vi "VisualizePmuResults.vi"() -> ()   [LabVIEW 2018, in "Visualization.lvlib" / "VisualizeAnalysis.lvclass"]
uses:
  VisualizeAnalysis.lvclass
  VisualizeBase/VisualizeBase_class/Requests/clUserEventType.ctl
  <vilib>/event_ctls.llb/usereventprio.ctl
  <vilib>/Utility/file.llb/Read From Spreadsheet File (DBL).vi
  <vilib>/Utility/error.llb/Error Cluster From Error Code.vi
  <vilib>/ErrorRing/Error Ring.xnode
  VisualizeBase/VisualizeBase_class/VisualizeBase.lvclass
  <userlib>/NIST/NISTErrorLib/NISTErrorLib.lvlib
  Analysis/AnalysisModule/AnalysisModule.lvlib
panel:
  in  "btnReset":bool
  in  "btnClear":bool
  in  "Pause":bool
  out "Data from file":dbl[][](array[numeric])
  in  "btnOpen":bool
  out "RFE":dbl(graph)
  out "FE":dbl(graph)
  out "Data real time":dbl[](array[numeric])
  out "TVE":cluster{timestamp[], dbl[]}[](graph)
  in  "QueName":string="AnalVisQue"
  out "ErrorArray":errorcluster[](array[cluster])
  in  "btnStop":bool
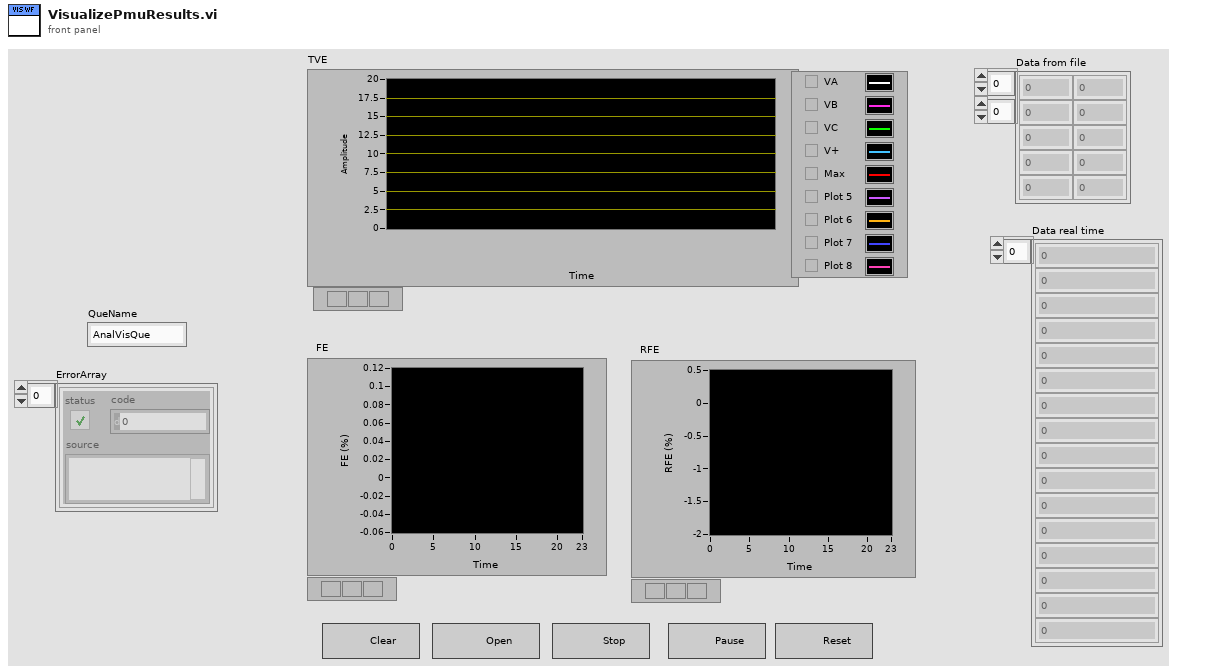
[diagram p1: front panel]
types:
  T1 = typedef "Visualization.lvlib/VisualizeBase.lvclass/clRequestEvents.ctl" = cluster{"StopRequest":refnum<user-event>, "ResetRequest":refnum<user-event>}
  T2 = typedef "AnalysisModule.lvlib/clBroadcastEvents.ctl" = cluster{"DidInit":refnum<user-event>, "StatusUpdate":refnum<user-event>, "ErrorReport":refnum<user-event>, "DidStop":refnum<user-event>, "PathToINI":refnum<user-event>, "Config":refnum<user-event>, "ResultReport":refnum<user-event>, "FunctionClass":refnum<user-event>}
  T3 = typedef "Visualization.lvlib/VisualizeBase.lvclass/clUserEventType.ctl" = cluster{"BusIndex":i8, "Data":variant}
  T4 = typedef "usereventprio.ctl" = enum32{"high priority", "normal priority"}
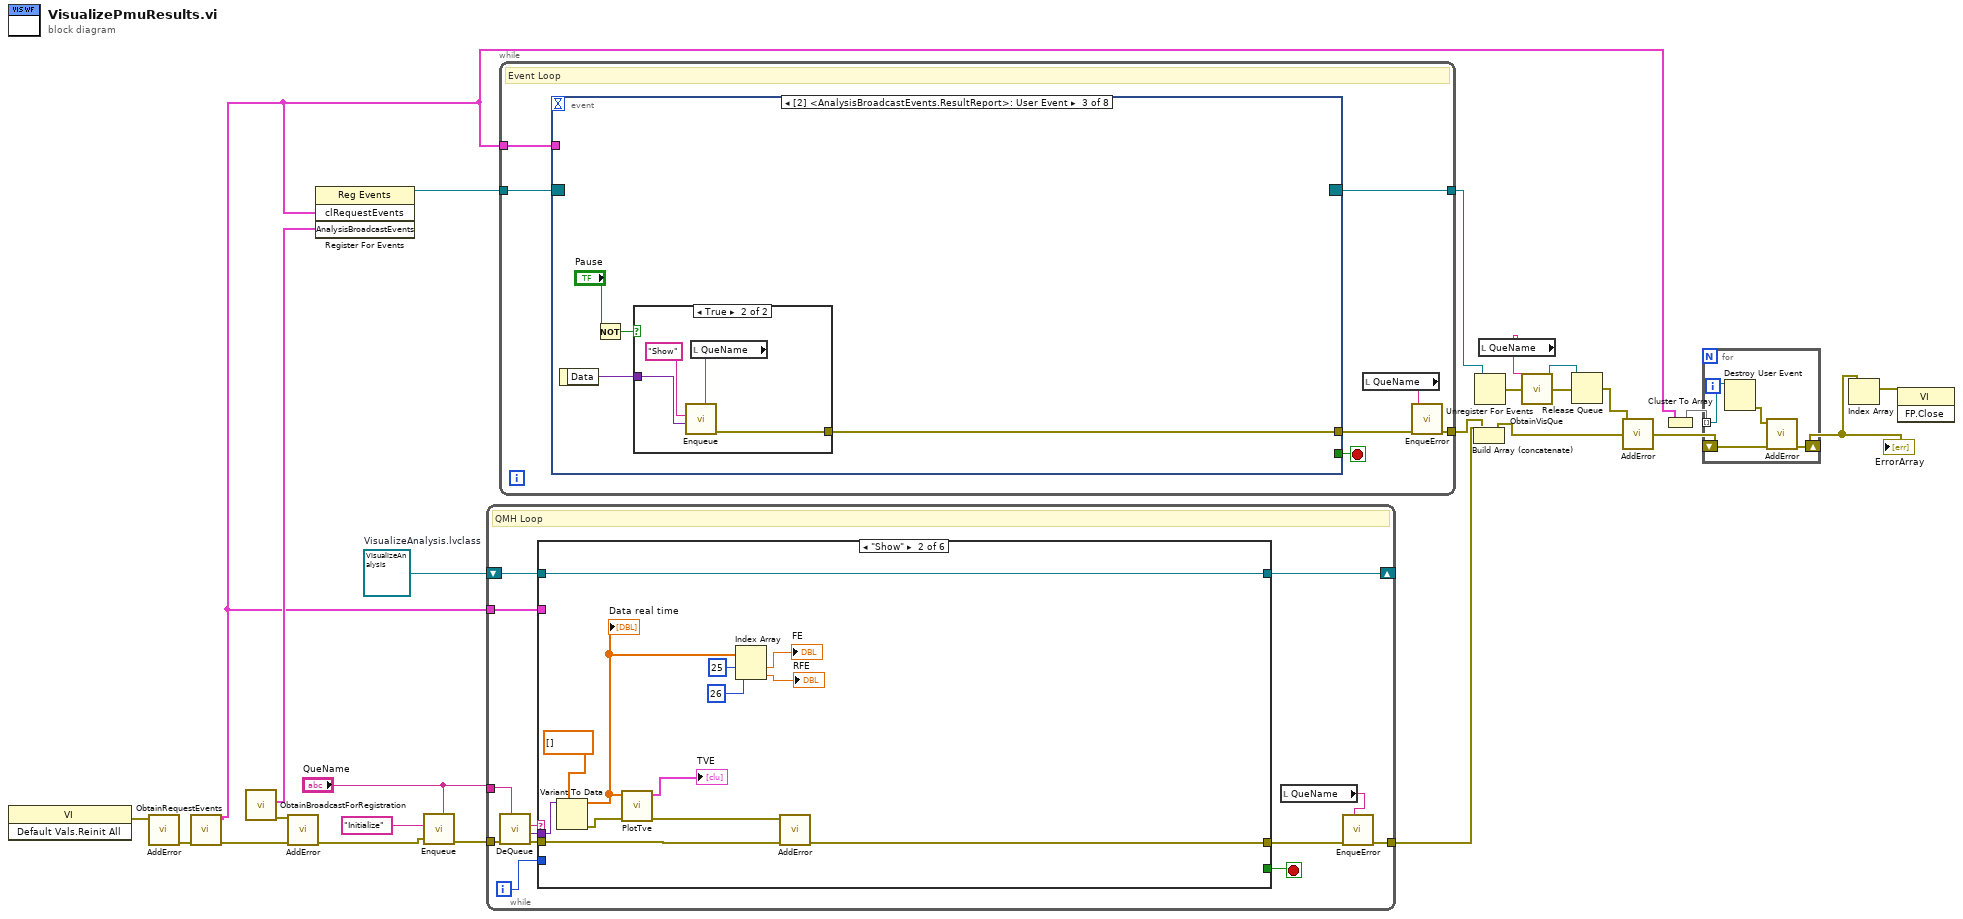
[diagram p0: block diagram]
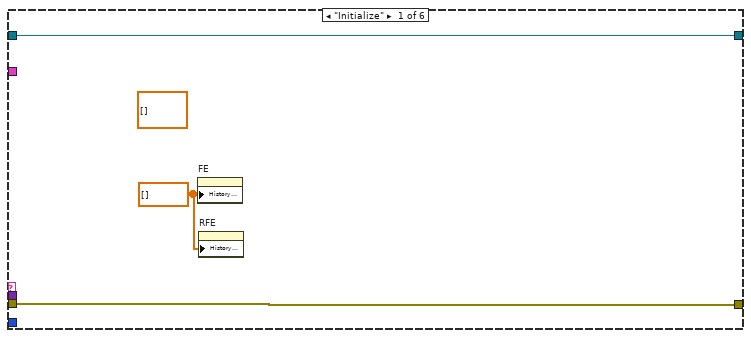
[diagram p2: hidden frame]
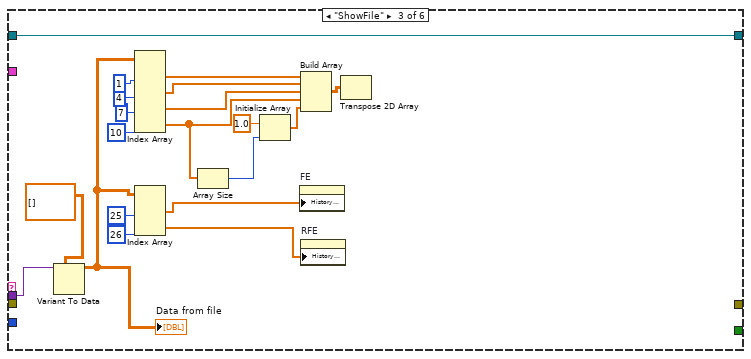
[diagram p3: hidden frame]
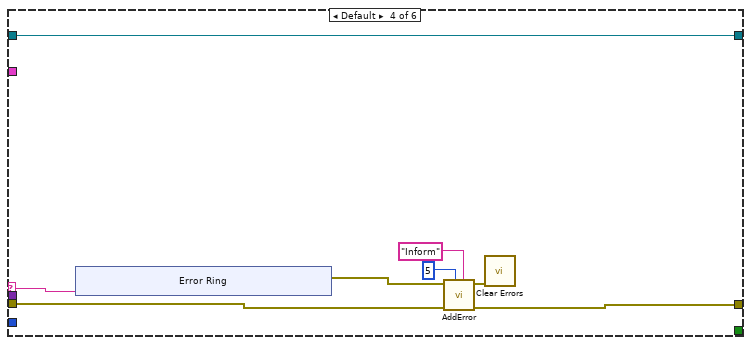
[diagram p4: hidden frame]
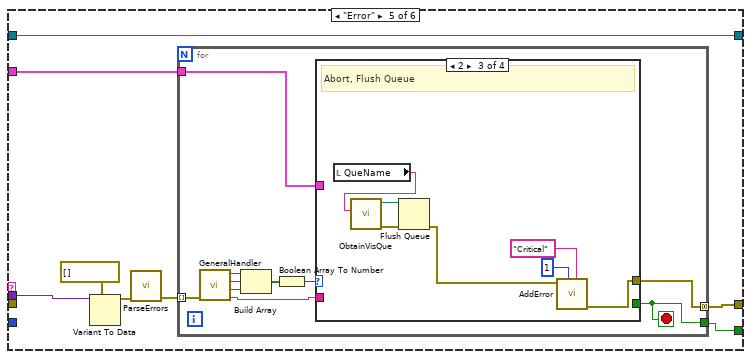
[diagram p5: hidden frame]
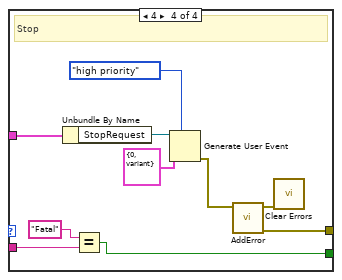
[diagram p8: hidden frame]
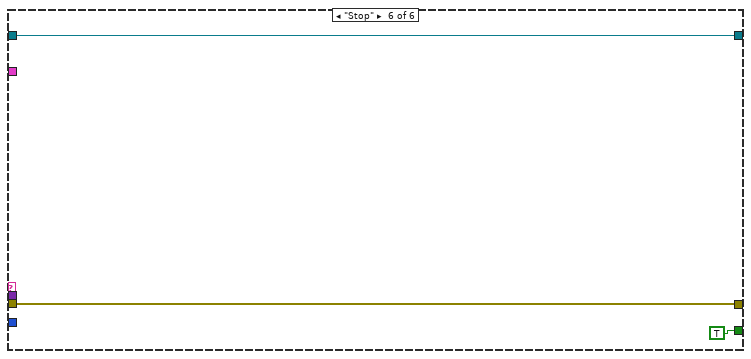
[diagram p9: hidden frame]
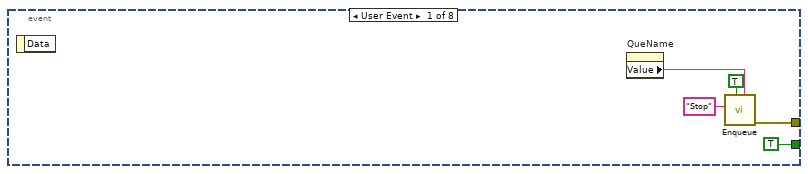
[diagram p10: hidden frame]
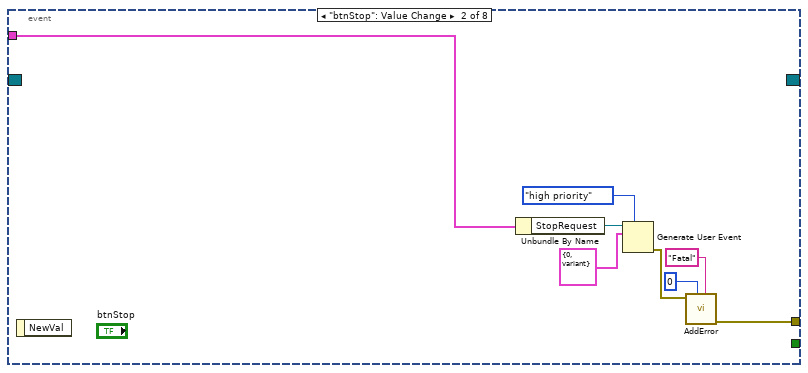
[diagram p11: hidden frame]
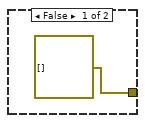
[diagram p12: hidden frame]
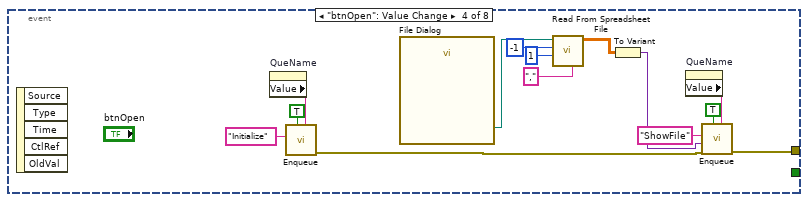
[diagram p13: hidden frame]
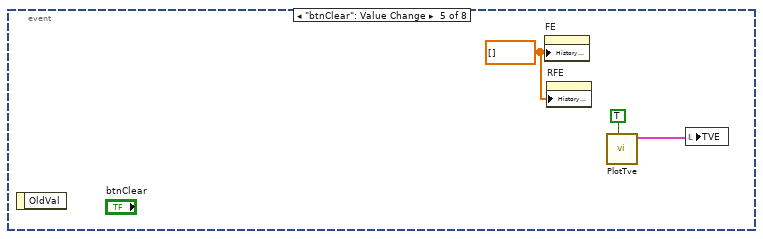
[diagram p14: hidden frame]
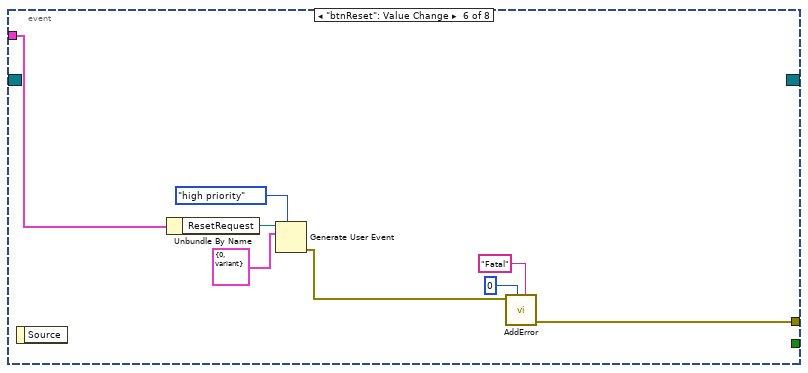
[diagram p15: hidden frame]
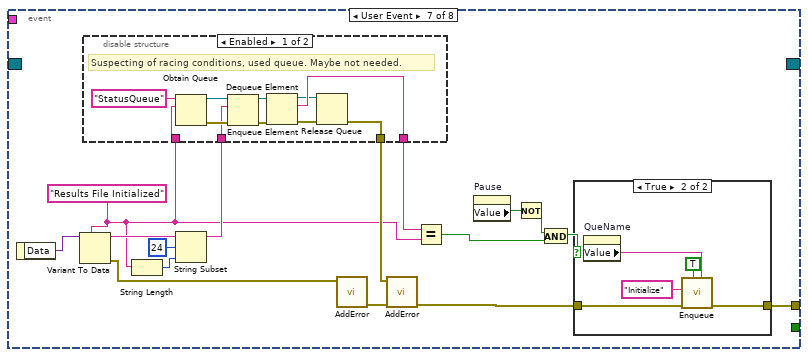
[diagram p16: hidden frame]
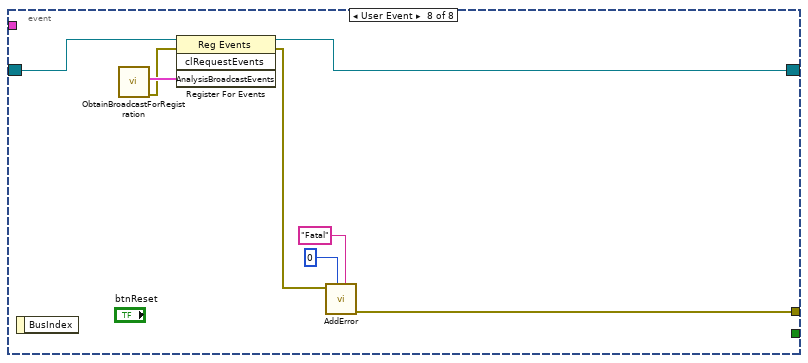
[diagram p19: hidden frame]
diagram:
  w14 = refnum<class "VisualizeAnalysis.lvclass"> refnum  # VisualizeAnalysis.lvclass
  n1 = invoke class="VI" method="Default Vals.Reinit All"() -> (error out=w21:errorcluster)  [unwired: 3 in, 2 out]
  n2 = call <userlib>:"AddError.vi"("error in (no error)"=w21) -> ("ErrorArray"=w20:errorcluster[])  [unwired: 9 in, 1 out]
  n3 = call "ObtainRequestEvents.vi"("Error"=w20) -> ("Error"=w18:errorcluster[], "clRequestEvents"=w1:T1)  [unwired: 9 in]
  n4 = call "ObtainBroadcastForRegistration.vi"() -> ("error out"=w16:errorcluster, "AnalysisBroadcastEvents"=w19:T2)  [unwired: 10 in]
  n5 = call <userlib>:"AddError.vi"("ErrorArray"=w18, "error in (no error)"=w16) -> ("ErrorArray"=w17:errorcluster[])  [unwired: 8 in, 1 out]
  n6 = register-events(w1, w19) -> (reference out=w13:refnum<event-registration>)  [unwired: 2 in, 1 out]
  n7 = call "Enqueue.vi"("QueName"="QueName", "Error"=w17, "Message"="Initialize") -> ("Error"=w24:errorcluster[])  [unwired: 8 in]
  n8 = while {
    tunnel: w24 -> [w38]
    tunnel: [w32] -> w23
    tunnel: "QueName" -> [w30]
    shift-right: [w29] -> _
    shift-left: w14 -> [w28]
    tunnel: w1 -> [w27]
    i -> [w26]
    stop <- w33 stop-if-true
    # "QMH Loop"
    n9 = call "DeQueue.vi"("QueName"=w30, "Error"=w38) -> ("Error"=w35:errorcluster[], "Data"=w36:variant, "Message"=w37:string)  [unwired: 7 in]
    n10 = case shown="\"Show\"" w37 {
      selector: w37 -> [_ _ _ w82 _ _]
      tunnel: w36 -> [_ w53 w74 _ w97 _]
      tunnel: w35 -> [w41 w48 _ w80 _ w126]
      tunnel: [w41 w47 _ w79 w93 w126] -> w34
      tunnel: [_ _ _ _ w92 TRUE] -> w33
      tunnel: w28 -> [w40 w54 w72 w75 w91 w125]
      tunnel: [w40 w54 w72 w75 w91 w125] -> w29
      tunnel: w27 -> [_ _ _ _ w90 _]
      tunnel: w26 -> [_ _ _ _ _ _]
      frame "Initialize" {
        w39 = dbl[] [] ("History Data")
        (unwired) dbl[][] [] ("History Data")
        n11 = property on="FE" class="WFChart (strict)"("History Data"=w39) -> ()  [unwired: 2 in, 2 out]
        n12 = property on="RFE" class="WFChart (strict)"("History Data"=w39) -> ()  [unwired: 2 in, 2 out]
      }
      frame "Show" {
        n13 = Variant To Data(type=dbl[] [], Variant=w53) -> (data=w44:dbl[], error out=w46:errorcluster)  [unwired: 1 in]
        "Data real time" <- w44
        n14 = call "PlotTve.vi"("error in (no error)"=w46, "Data real time"=w44) -> ("error out"=w45:errorcluster, "TVE"=→"TVE":cluster{timestamp[], dbl[]}[])  [unwired: 8 in]
        n15 = Index Array(array=w44, index #1=25 ("index"), index #2=26 ("index")) -> (element #1=→"FE":dbl, element #2=→"RFE":dbl)
        n16 = call <userlib>:"AddError.vi"("ErrorArray"=w48, "error in (no error)"=w45) -> ("ErrorArray"=w47:errorcluster[])  [unwired: 8 in, 1 out]
      }
      frame "ShowFile" {
        n17 = Variant To Data(type=dbl[][] [], Variant=w74) -> (data=w63:dbl[][])  [unwired: 1 in, 1 out]
        "Data from file" <- w63
        n18 = Index Array(array=w63, index (col) #1=1 ("disabled index (col)"), index (col) #2=4 ("index (col)"), index (col) #3=7 ("index (col)"), index (col) #4=10 ("index (col)")) -> (element #1=w67:dbl[], element #2=w66:dbl[], element #3=w65:dbl[], element #4=w58:dbl[])  [unwired: 4 in]
        n19 = Index Array(array=w63, index (col) #1=25 ("disabled index (col)"), index (col) #2=26 ("index (col)")) -> (element #1=w60:dbl[], element #2=w59:dbl[])  [unwired: 2 in]
        n20 = Array Size(array=w58) -> (size(s)=w57:i32)
        n21 = Initialize Array(1.0 ("element"), w57) -> (w55:dbl[])
        n22 = property on="FE" class="WFChart (strict)"("History Data"=w60) -> ()  [unwired: 2 in, 2 out]
        n23 = Build Array(w67, w66, w65, w58, w55) -> (w64:dbl[][])
        n24 = property on="RFE" class="WFChart (strict)"("History Data"=w59) -> ()  [unwired: 2 in, 2 out]
        n25 = Transpose 2D Array(2D array=w64) -> ()  [unwired: 1 out]
      }
      frame Default {
        n26 = xnode "Error Ring"("parameter 0"=w82) -> ("error out"=w81:errorcluster)
        n27 = call <userlib>:"AddError.vi"("Severity"="Inform" ("String"), "Priority"=u8 5, "ErrorArray"=w80, "error in (no error)"=w81) -> ("ErrorArray"=w79:errorcluster[], "error out"=w78:errorcluster)  [unwired: 6 in]
        n28 = call <vilib>:"Clear Errors.vi"("error in (no error)"=w78) -> ()  [unwired: 5 in, 2 out]
      }
      frame "Error" {
        n29 = Variant To Data(type=errorcluster[] [], Variant=w97) -> (data=w95:errorcluster[])  [unwired: 1 in, 1 out]
        n30 = call <userlib>:"ParseErrors.vi"("ErrorArray"=w95) -> ("ErrorArray"=w94:errorcluster[])  [unwired: 8 in, 2 out]
        n31 = for {
          tunnel: w94 -> [w107] mode=indexing
          tunnel: [w101] -> w93 mode=concatenating
          tunnel: [w99] -> w92
          tunnel: w90 -> [w98]
          stop <- w99 stop-if-true
          n32 = call <userlib>:"GeneralHandler.vi"("error in (no error)"=w107) -> ("Severity"=w100:string, "Stop"=w104:bool, "Abort"=w105:bool, "Continue"=w106:bool)  [unwired: 7 in]
          n33 = Build Array(w106, w105, w104) -> (w103:bool[])
          n34 = Boolean Array To Number(Boolean array=w103) -> (number=w102:u32)
          n35 = case shown="2" w102 {
            tunnel: [_ _ w112 w123] -> w101
            tunnel: w100 -> [_ _ _ w118]
            tunnel: [_ _ _ w116] -> w99
            tunnel: w98 -> [_ _ _ w115]
            frame 0, Default {
              # "No Dialog"
            }
            frame 1 {
              # "Continue"
            }
            frame 2 {
              # "Abort, Flush Queue"
              n36 = local read "QueName"() -> (w108:string)
              n37 = call "ObtainVisQue.vi"("QueName"=w108) -> ("error out"=w114:errorcluster, "queue out"=w113:refnum<queue>)  [unwired: 9 in]
              n38 = Flush Queue(queue=w113, error in (no error)=w114) -> (error out=w111:errorcluster)  [unwired: 2 out]
              n39 = call <userlib>:"AddError.vi"("Severity"="Critical" ("String"), "Priority"=u8 1, "error in (no error)"=w111) -> ("ErrorArray"=w112:errorcluster[])  [unwired: 7 in, 1 out]
            }
            frame 4 {
              # "Stop"
              n40 = Unbundle By Name(w115) -> ("StopRequest"=w124:refnum<user-event>)
              n41 = Equal?(x="Fatal", y=w118) -> (x = y?=w116:bool)
              n42 = Generate User Event(priority (normal)=usereventprio."high priority", user event=w124, event data cluster=T3 {"BusIndex"=0, "Data"=variant} ("event data")) -> (error out=w122:errorcluster)  [unwired: 1 in, 1 out]
              n43 = call <userlib>:"AddError.vi"("error in (no error)"=w122) -> ("ErrorArray"=w123:errorcluster[], "error out"=w119:errorcluster)  [unwired: 9 in]
              n44 = call <vilib>:"Clear Errors.vi"("error in (no error)"=w119) -> ()  [unwired: 5 in, 2 out]
            }
          }
        }
      }
      frame "Stop" {
      }
    }
    n45 = local read "QueName"() -> (w31:string)
    n46 = call "EnqueError.vi"("QueName"=w31, "Error"=w34) -> ("Error"=w32:errorcluster[])  [unwired: 9 in]
  }
  n47 = while {
    tunnel: [w132] -> w22
    tunnel: w13 -> [w130]
    tunnel: [w129] -> w7
    tunnel: w1 -> [w128]
    stop <- w134 stop-if-true
    # "Event Loop"
    n48 = event shown="[2] <AnalysisBroadcastEvents.ResultReport>: User Event" {
      selector: w130 -> [_ _ _ _ _ _ _ w216]
      dyn-events: [_ _ _ _ _ _ _ w221] -> w129
      timeout: _ -> [_ _ _ _ _ _ _ _]
      tunnel: [TRUE _ _ _ _ _ _ _] -> w134
      tunnel: [w138 w145 w150 w165 _ w174 w196 w217] -> w133
      tunnel: w128 -> [_ w140 _ _ _ w175 _ _]
      event User Event {
        n49 = event-data() -> ()  [unwired: 1 in, 1 out]
        n50 = property on="QueName" class="Str"() -> ("Value"=w135:string)  [unwired: 2 in, 2 out]
        n51 = call "Enqueue.vi"("QueName"=w135, "Priority? (F)"=TRUE, "Message"="Stop") -> ("Error"=w138:errorcluster[])  [unwired: 8 in]
      }
      event "btnStop": Value Change {
        n52 = event-data() -> ()  [unwired: 1 in, 1 out]
        n53 = Unbundle By Name(w140) -> ("StopRequest"=w146:refnum<user-event>)
        n54 = Generate User Event(priority (normal)=usereventprio."high priority", user event=w146, event data cluster=T3 {"BusIndex"=0, "Data"=variant} ("event data")) -> (error out=w147:errorcluster)  [unwired: 1 in, 1 out]
        n55 = call <userlib>:"AddError.vi"("Severity"="Fatal" ("String"), "Priority"=u8 0, "error in (no error)"=w147) -> ("ErrorArray"=w145:errorcluster[])  [unwired: 7 in, 1 out]
      }
      event User Event {
        n56 = event-data() -> ("Data"=w151:variant)  [unwired: 1 in]
        n57 = Not(x="Pause") -> (.not. x?=w148:bool)
        n58 = case shown="True" w148 {
          tunnel: w151 -> [_ w155]
          tunnel: [errorcluster[] [] ("Error") w154] -> w150
          frame False {
          }
          frame True {
            n59 = local read "QueName"() -> (w156:string)
            n60 = call "Enqueue.vi"("QueName"=w156, "Data"=w155, "Message"="Show") -> ("Error"=w154:errorcluster[])  [unwired: 8 in]
          }
        }
      }
      event "btnOpen": Value Change {
        n61 = event-data() -> ()  [unwired: 1 in, 5 out]
        n62 = property on="QueName" class="Str"() -> ("Value"=w162:string)  [unwired: 2 in, 2 out]
        n63 = call "Enqueue.vi"("QueName"=w162, "Priority? (F)"=TRUE, "Message"="Initialize") -> ("Error"=w159:errorcluster[])  [unwired: 8 in]
        n64 = call "File Dialog"() -> ("selected path"=w170:path)  [unwired: 12 in, 3 out]
        n65 = call-poly <vilib>:"Read From Spreadsheet File.vi"("delimiter (\\t)"="," ("delimiter (\\t)"), "start of read offset (chars.:0)"=1, "number of rows (all:-1)"=-1, "file path (dialog if empty)"=w170) -> ("all rows"=w164:dbl[][])  [unwired: 3 in, 4 out]
        n66 = To Variant(anything=w164) -> (Variant=w163:variant)
        n67 = property on="QueName" class="Str"() -> ("Value"=w166:string)  [unwired: 2 in, 2 out]
        n68 = call "Enqueue.vi"("QueName"=w166, "Priority? (F)"=TRUE, "Error"=w159, "Data"=w163, "Message"="ShowFile") -> ("Error"=w165:errorcluster[])  [unwired: 6 in]
      }
      event "btnClear": Value Change {
        w171 = dbl[] [] ("History Data")
        n69 = event-data() -> ()  [unwired: 1 in, 1 out]
        n70 = property on="FE" class="WFChart (strict)"("History Data"=w171) -> ()  [unwired: 2 in, 2 out]
        n71 = property on="RFE" class="WFChart (strict)"("History Data"=w171) -> ()  [unwired: 2 in, 2 out]
        n72 = call "PlotTve.vi"("Clear? (f)"=TRUE) -> ("TVE"=w172:cluster{timestamp[], dbl[]}[])  [unwired: 9 in, 1 out]
        n73 = local write "TVE"(w172) -> ()
      }
      event "btnReset": Value Change {
        n74 = event-data() -> ()  [unwired: 1 in, 1 out]
        n75 = Unbundle By Name(w175) -> ("ResetRequest"=w176:refnum<user-event>)
        n76 = Generate User Event(priority (normal)=usereventprio."high priority", user event=w176, event data cluster=T3 {"BusIndex"=0, "Data"=variant} ("event data")) -> (error out=w179:errorcluster)  [unwired: 1 in, 1 out]
        n77 = call <userlib>:"AddError.vi"("Severity"="Fatal", "Priority"=u8 0, "error in (no error)"=w179) -> ("ErrorArray"=w174:errorcluster[])  [unwired: 7 in, 1 out]
      }
      event User Event {
        w186 = "Results File Initialized" ("Status")
        n78 = event-data() -> ("Data"=w197:variant)  [unwired: 1 in]
        n79 = Variant To Data(type=w186, Variant=w197) -> (data=w194:string, error out=w191:errorcluster)  [unwired: 1 in]
        n80 = String Length(string=w186) -> (length=w187:i32)
        n81 = String Subset(string=w194, offset (0)=24, length (rest)=w187) -> (substring=w189:string)
        n82 = disable-structure shown="Enabled" {
          disable-tunnel: [w201 w209] -> w193
          disable-tunnel: [w198 _] -> w190
          disable-tunnel: w189 -> [w203 w209]
          disable-tunnel: w186 -> [w202 _]
          frame Enabled {
            # "Suspecting of racing conditions, used queue. Maybe not needed."
            n83 = Obtain Queue(name (unnamed)="StatusQueue", element data type=w202) -> (queue out=w207:refnum<queue>, error out=w205:errorcluster)  [unwired: 3 in, 1 out]
            n84 = Enqueue Element(queue=w207, element=w203, error in (no error)=w205) -> (queue out=w206:refnum<queue>, error out=w204:errorcluster)  [unwired: 1 in, 1 out]
            n85 = Dequeue Element(queue=w206, error in (no error)=w204) -> (queue out=w200:refnum<queue>, element=w201:string, error out=w199:errorcluster)  [unwired: 1 in, 1 out]
            n86 = Release Queue(queue=w200, error in (no error)=w199) -> (error out=w198:errorcluster)  [unwired: 1 in, 2 out]
          }
          frame Disabled {
          }
        }
        n87 = call <userlib>:"AddError.vi"("error in (no error)"=w191) -> ("ErrorArray"=w192:errorcluster[])  [unwired: 9 in, 1 out]
        n88 = call <userlib>:"AddError.vi"("ErrorArray"=w192, "error in (no error)"=w190) -> ("ErrorArray"=w195:errorcluster[])  [unwired: 8 in, 1 out]
        n89 = Equal?(x=w193, y=w186) -> (x = y?=w184:bool)
        n90 = property on="Pause" class="Bool (strict)"() -> ("Value"=w183:bool)  [unwired: 2 in, 2 out]
        n91 = Not(x=w183) -> (.not. x?=w182:bool)
        n92 = And(x=w182, y=w184) -> (x .and. y?=w185:bool)
        n93 = case shown="True" w185 {
          tunnel: [w210 w212] -> w196
          tunnel: w195 -> [w210 w211]
          frame False {
          }
          frame True {
            n94 = property on="QueName" class="Str"() -> ("Value"=w213:string)  [unwired: 2 in, 2 out]
            n95 = call "Enqueue.vi"("QueName"=w213, "Priority? (F)"=TRUE, "Error"=w211, "Message"="Initialize") -> ("Error"=w212:errorcluster[])  [unwired: 7 in]
          }
        }
      }
      event User Event {
        n96 = event-data() -> ()  [unwired: 1 in, 1 out]
        n97 = call "ObtainBroadcastForRegistration.vi"() -> ("error out"=w222:errorcluster, "AnalysisBroadcastEvents"=w223:T2)  [unwired: 10 in]
        n98 = register-events(reference=w216, error in=w222, w223) -> (reference out=w221:refnum<event-registration>, error out=w220:errorcluster)  [unwired: 1 in]
        n99 = call <userlib>:"AddError.vi"("Severity"="Fatal", "Priority"=u8 0, "error in (no error)"=w220) -> ("ErrorArray"=w217:errorcluster[])  [unwired: 7 in, 1 out]
      }
    }
    n100 = local read "QueName"() -> (w131:string)
    n101 = call "EnqueError.vi"("QueName"=w131, "Error"=w133) -> ("Error"=w132:errorcluster[])  [unwired: 9 in]
  }
  n102 = Build Array (concatenate)(w22, w23) -> (w6:errorcluster[])
  n103 = Unregister For Events(event registration refnum=w7) -> (error out=w9:errorcluster)  [unwired: 1 in]
  n104 = local read "QueName"() -> (w3:string)
  n105 = call "ObtainVisQue.vi"("error in (no error)"=w9, "QueName"=w3) -> ("error out"=w10:errorcluster, "queue out"=w11:refnum<queue>)  [unwired: 8 in]
  n106 = Release Queue(queue=w11, error in (no error)=w10) -> (error out=w12:errorcluster)  [unwired: 1 in, 2 out]
  n107 = call <userlib>:"AddError.vi"("ErrorArray"=w6, "error in (no error)"=w12) -> ("ErrorArray"=w2:errorcluster[])  [unwired: 8 in, 1 out]
  n108 = Cluster To Array(cluster=w1) -> (array=w8:refnum<user-event>[])
  n109 = for {
    tunnel: w8 -> [w227] mode=indexing
    shift-right: [w226] -> w5
    shift-left: w2 -> [w225]
    n110 = Destroy User Event(user event=w227) -> (error out=w224:errorcluster)  [unwired: 1 in]
    n111 = call <userlib>:"AddError.vi"("ErrorArray"=w225, "error in (no error)"=w224) -> ("ErrorArray"=w226:errorcluster[])  [unwired: 8 in, 1 out]
  }
  "ErrorArray" <- w5
  n112 = Index Array(array=w5) -> (element=w4:errorcluster)  [unwired: 1 in]
  n113 = invoke class="VI" method="FP.Close"(error in=w4) -> ()  [unwired: 2 in, 3 out]
